vi "app global state.vi"(0 "action":T4=enum."set cluster", 1 "magnet polar":T3, 2 "field ramping":bool, 3 "vna sweeping":bool, 4 "log line to append":string, 5 "initial value":T5 {"Current Magnetic Field\n(430 TCP reading)"."phi (deg)" format="%#_3g"}, 6 "measurement finished":bool, 7 "current sweep":T1, 8 "field was reached":bool, 9 "Current Magnetic Field\n(430 TCP reading)":cluster{"magnitude (T)":dbl, "phi (deg)":dbl} {"phi (deg)" format="%#_3g"}) -> (19 "global state":T5 {"Current Magnetic Field\n(430 TCP reading)"."phi (deg)" format="%#_3g"})   [LabVIEW 2013]
uses:
  app global state control.ctl
  devices/magnet/magnet polar field.ctl
  measurement/measconfig cluster.ctl
  measurement/measurement sweep parameter.ctl
  app global state actions.ctl
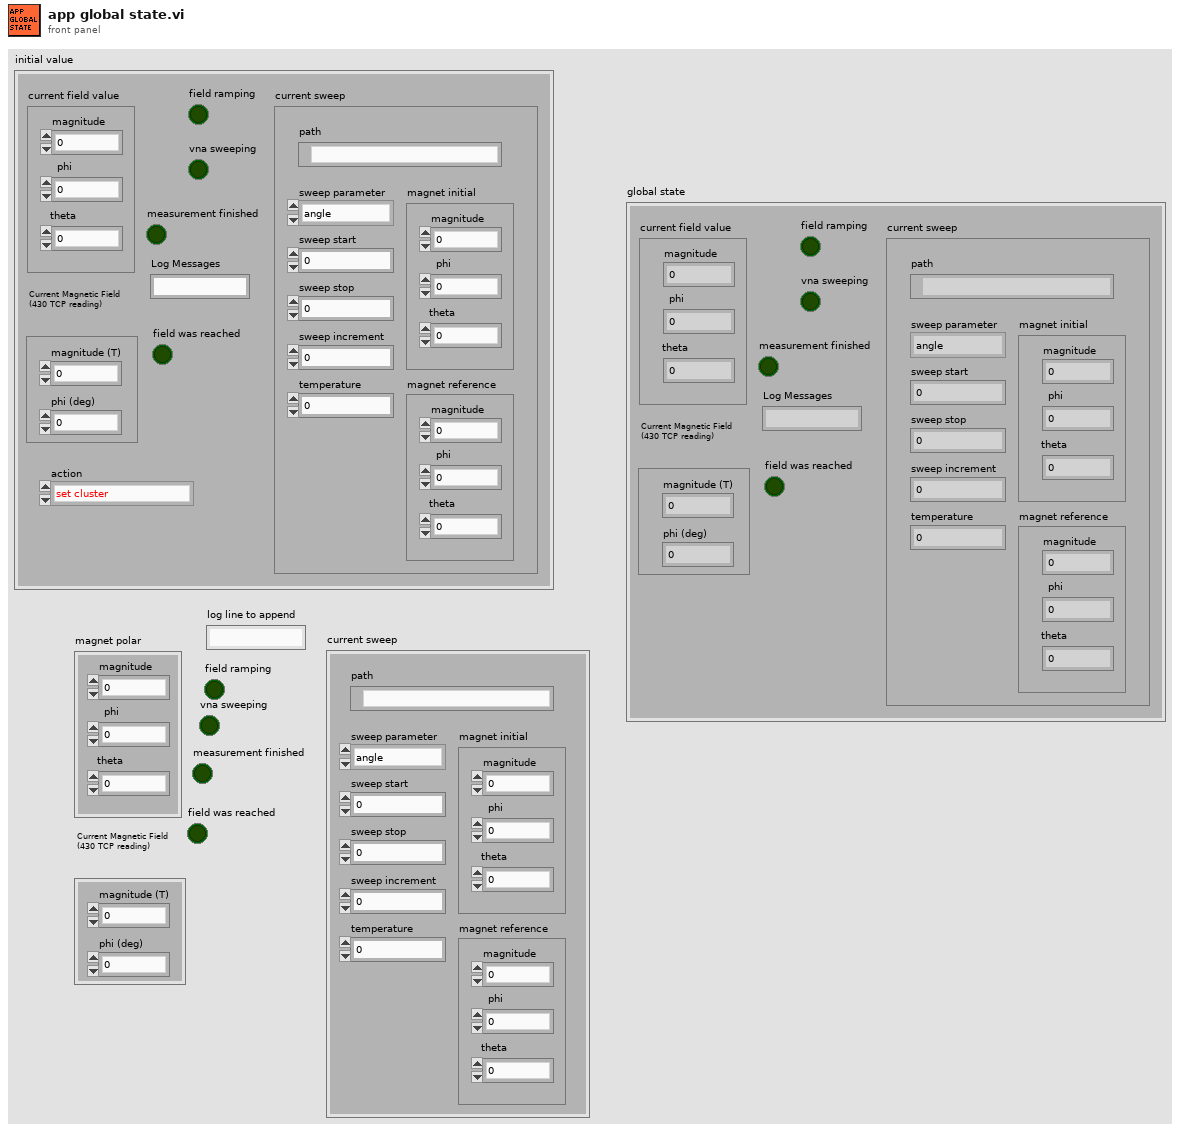
[diagram p1: front panel]
types:
  T1 = typedef "measconfig cluster.ctl" = cluster{"sweep parameter":T2, "sweep start":dbl, "sweep stop":dbl, "sweep increment":dbl, "temperature":dbl, "path":path, "magnet initial":T3, "magnet reference":T3}
  T2 = typedef "measurement sweep parameter.ctl" = enum16{"angle", "magnetic field"}
  T3 = typedef "magnet polar field.ctl" = cluster{"magnitude":dbl, "phi":dbl, "theta":dbl}
  T4 = typedef "app global state actions.ctl" = enum16{"set field reached", "get cluster", "set cluster", "set current sweep", "set field value", "set 430 TCP reading", "set ramping", "set sweeping", "append log", "clear log", "set finished"}
  T5 = typedef "app global state control.ctl" = cluster{"current field value":T3, "field ramping":bool, "vna sweeping":bool, "Log Messages":string, "current sweep":T1, "measurement finished":bool, "Current Magnetic Field\n(430 TCP reading)":cluster{"magnitude (T)":dbl, "phi (deg)":dbl}, "field was reached":bool}
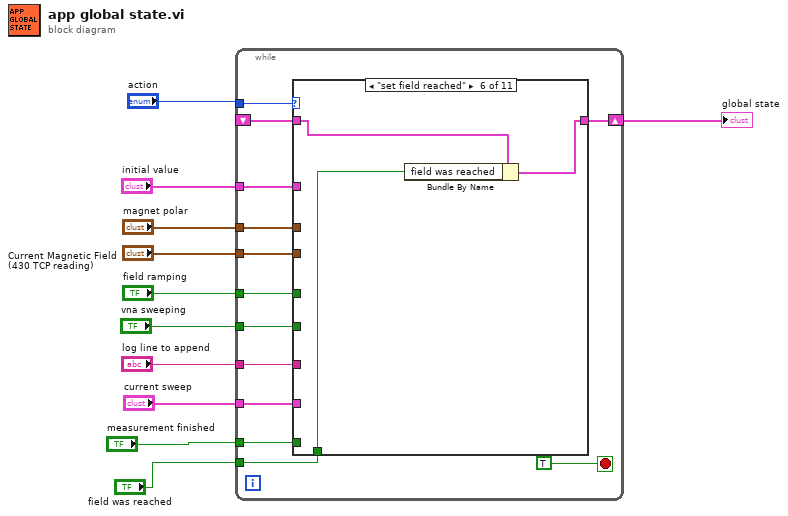
[diagram p0: block diagram]
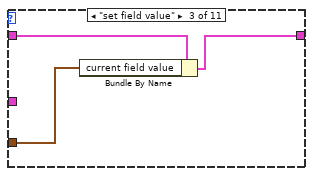
[diagram p4: hidden frame]
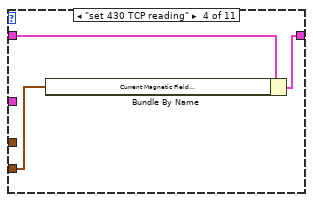
[diagram p5: hidden frame]
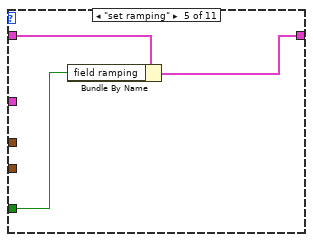
[diagram p6: hidden frame]
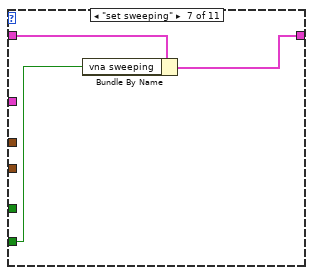
[diagram p7: hidden frame]
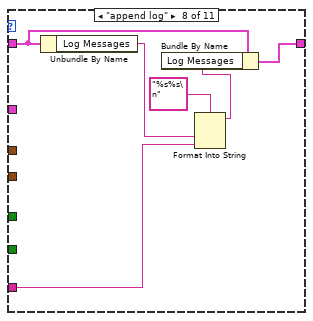
[diagram p8: hidden frame]
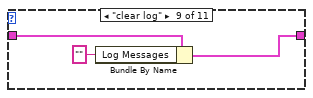
[diagram p9: hidden frame]
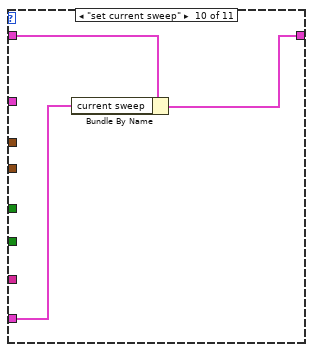
[diagram p10: hidden frame]
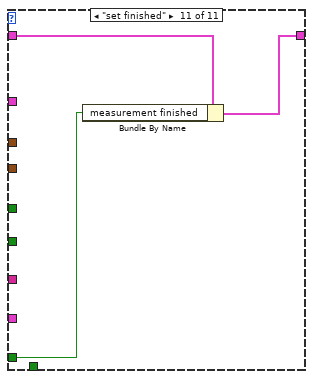
[diagram p11: hidden frame]
diagram:
  n1 = while {
    tunnel: "action" -> [w23]
    shift-right: [w21] -> w11
    shift-left: _ -> [w22]
    tunnel: "initial value" -> [w20]
    tunnel: "magnet polar" -> [w19]
    tunnel: "field ramping" -> [w18]
    tunnel: "log line to append" -> [w17]
    tunnel: "current sweep" -> [w16]
    tunnel: "measurement finished" -> [w15]
    tunnel: "vna sweeping" -> [w14]
    tunnel: "Current Magnetic Field\n(430 TCP reading)" -> [w13]
    tunnel: "field was reached" -> [w12]
    stop <- TRUE stop-if-true
    n2 = case shown="\"set field reached\"" w23 {
      tunnel: w22 -> [_ w26 w29 w31 w33 w38 w40 w47 w50 w53 w56]
      tunnel: [w25 w26 w28 w32 w34 w36 w41 w42 w49 w51 w55] -> w21
      tunnel: w20 -> [w25 _ _ _ _ _ _ _ _ _ _]
      tunnel: w19 -> [_ _ w27 _ _ _ _ _ _ _ _]
      tunnel: w18 -> [_ _ _ _ w35 _ _ _ _ _ _]
      tunnel: w17 -> [_ _ _ _ _ _ _ w44 _ _ _]
      tunnel: w16 -> [_ _ _ _ _ _ _ _ _ w52 _]
      tunnel: w15 -> [_ _ _ _ _ _ _ _ _ _ w54]
      tunnel: w14 -> [_ _ _ _ _ _ w39 _ _ _ _]
      tunnel: w13 -> [_ _ _ w30 _ _ _ _ _ _ _]
      tunnel: w12 -> [_ _ _ _ _ w37 _ _ _ _ _]
      frame "set cluster", Default {
      }
      frame "get cluster" {
      }
      frame "set field value" {
        n3 = Bundle By Name(cluster=w29, "current field value"=w27) -> (w28:T5)
      }
      frame "set 430 TCP reading" {
        n4 = Bundle By Name(cluster=w31, "Current Magnetic Field\n(430 TCP reading)"=w30) -> (w32:T5)
      }
      frame "set ramping" {
        n5 = Bundle By Name(cluster=w33, "field ramping"=w35) -> (w34:T5)
      }
      frame "set field reached" {
        n6 = Bundle By Name(cluster=w38, "field was reached"=w37) -> (w36:T5)
      }
      frame "set sweeping" {
        n7 = Bundle By Name(cluster=w40, "vna sweeping"=w39) -> (w41:T5)
      }
      frame "append log" {
        n8 = Unbundle By Name(w47) -> ("Log Messages"=w45:string)
        n9 = Format Into String(format string="%s%s\n", w45, w44) -> (resulting string=w43:string)  [unwired: 2 in, 1 out]
        n10 = Bundle By Name(cluster=w47, "Log Messages"=w43) -> (w42:T5)
      }
      frame "clear log" {
        n11 = Bundle By Name(cluster=w50, "Log Messages"="") -> (w49:T5)
      }
      frame "set current sweep" {
        n12 = Bundle By Name(cluster=w53, "current sweep"=w52) -> (w51:T5)
      }
      frame "set finished" {
        n13 = Bundle By Name(cluster=w56, "measurement finished"=w54) -> (w55:T5)
      }
    }
  }
  "global state" <- w11
